vi "przyciski.vi"(3 "Akcja":T2, 5 "Wejœcie":T1) -> (2 "Wyjœcie":T1)   [LabVIEW 2014]
uses:
  Akcja_kontrolki.ctl
  przyciskiVIs/Przyciski_zbior.ctl
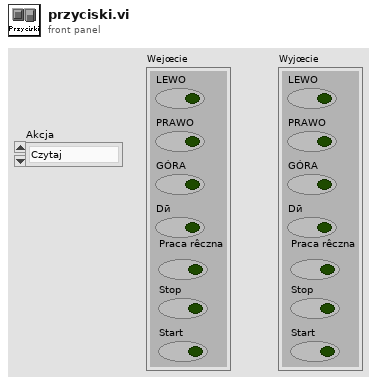
[diagram p1: front panel]
types:
  T1 = typedef "Przyciski_zbior.ctl" = cluster{"LEWO":bool, "PRAWO":bool, "GÓRA":bool, "Dӣ":bool, "Stop":bool, "Start":bool, "Praca rêczna":bool}
  T2 = typedef "Akcja_kontrolki.ctl" = enum16{"Czytaj", "Zapisz"}
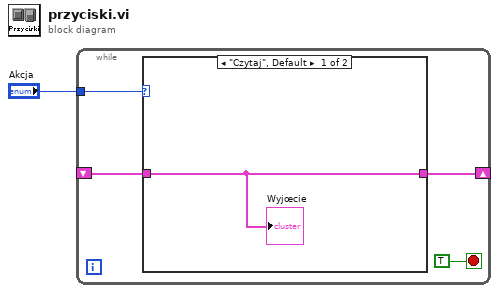
[diagram p0: block diagram]
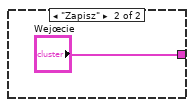
[diagram p2: hidden frame]
diagram:
  n1 = while {
    shift-right: [w3] -> _
    shift-left: _ -> [w2]
    tunnel: "Akcja" -> [w4]
    stop <- TRUE stop-if-true
    n2 = case shown="\"Czytaj\", Default" w4 {
      tunnel: [w6 "Wejœcie"] -> w3
      tunnel: w2 -> [w6 _]
      frame "Czytaj", Default {
        "Wyjœcie" <- w6
      }
      frame "Zapisz" {
      }
    }
  }
